vi "RTM - Add Packet.vi"() -> ()   [LabVIEW 2019, in "UDP-Custom-Device System Explorer.lvlib"]
uses:
  UDP-Custom-Device System Explorer.lvlib
  <vilib>/NI VeriStand/Custom Device Tools/Custom Device Utility Library/Custom Device Utility Library.lvlib
  <vilib>/NI VeriStand/Custom Device API/Custom Device API.lvlib
  Property Accessors/Shared Packet Accessors.lvlib
panel:
  in  "Buffered?":bool
  in  "Cancel Button":bool
  in  "OK Button":bool
  out "New Packet ID":i32
  in  "New Packet Name":string
  in  "Tag":string
  in  "Node Ptr":u64 format="%.0x"
  out "error out":errorcluster
  in  "error in (no error)":errorcluster
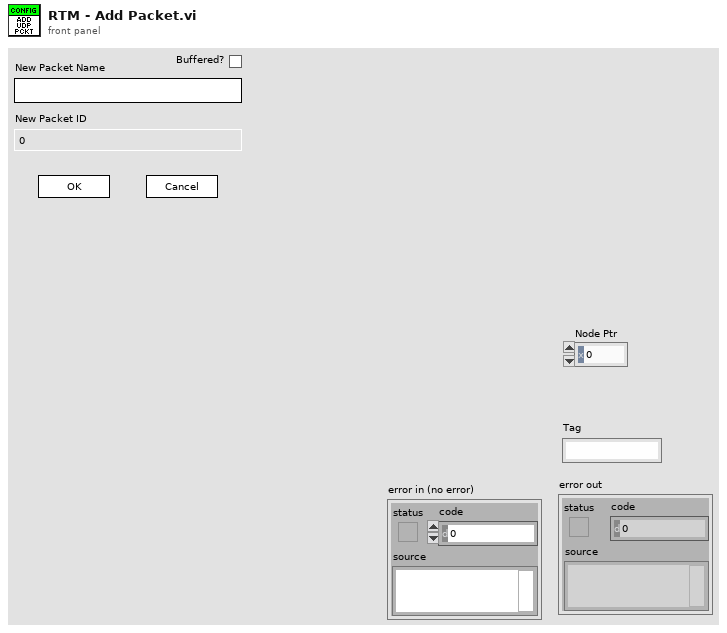
[diagram p1: front panel]
types:
  T1 = enum8{"Enabled", "Disabled", "Disabled and Grayed Out"}
  T2 = enum32{"Invalid", "Standard", "Closed", "Hidden", "Minimized", "Maximized"}
  T3 = typedef "Custom Device API.lvlib/Custom Device Item Ref.ctl" = u64
  T4 = typedef "UDP-Custom-Device System Explorer.lvlib/Packet Type.ctl" = enum16{"Transmit", "Receive", "Buffered Transmit", "Buffered Receive"}
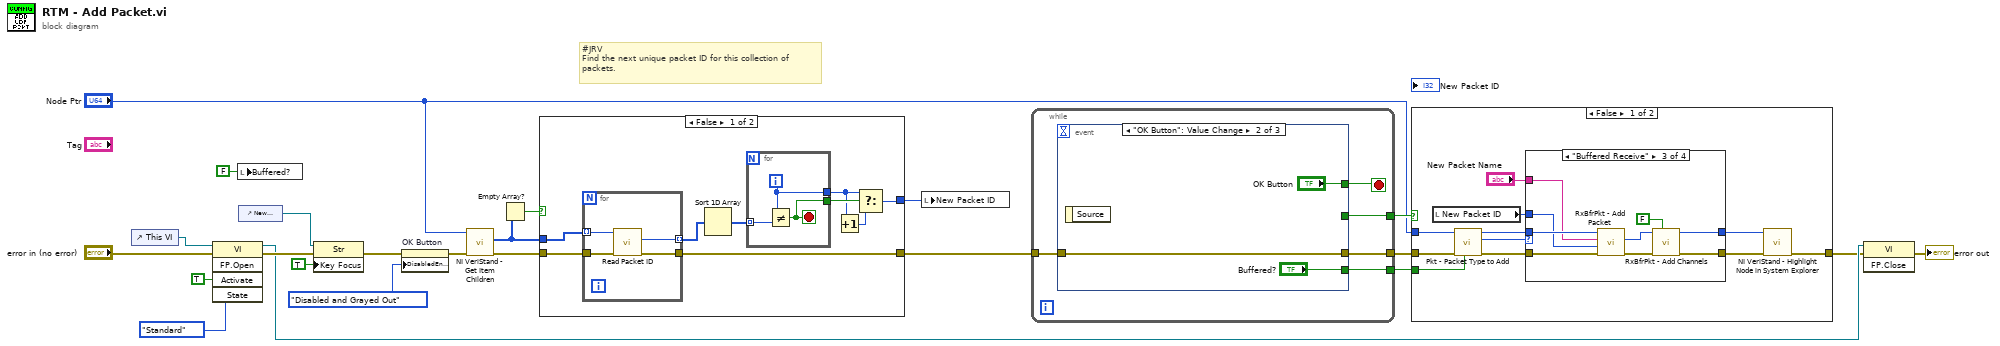
[diagram p0: block diagram]
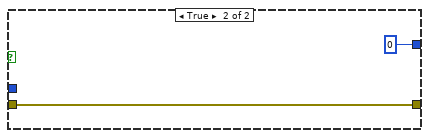
[diagram p2: hidden frame]
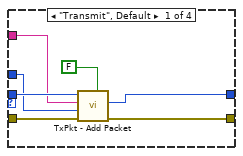
[diagram p3: hidden frame]
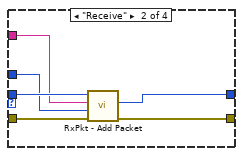
[diagram p4: hidden frame]
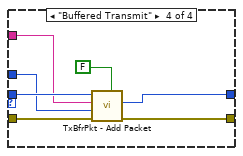
[diagram p5: hidden frame]
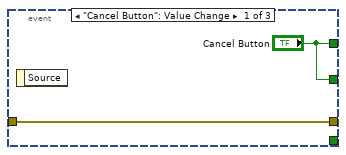
[diagram p7: hidden frame]
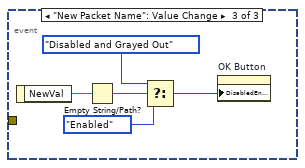
[diagram p8: hidden frame]
diagram:
  # "#JRV\nFind the next unique packet ID for this collection of\npackets."
  n1 = control-ref of="This VI"() -> (w23:refnum<vi>)
  n2 = invoke class="VI" method="FP.Open"(reference=w23, error in="error in (no error)", "Activate"=TRUE ("Activate?"), "State"=T2."Standard") -> (reference out=w15:refnum<vi>, error out=w19:errorcluster)  [unwired: 1 in, 3 out]
  n3 = local write "Buffered?"(FALSE ("Buffered?")) -> ()
  n4 = control-ref of="New Packet Name"() -> (w13:refnum<vi>)
  n5 = property class="Str"(reference=w13, error in=w19, "Key Focus"=TRUE) -> (error out=w4:errorcluster)  [unwired: 1 out]
  n6 = property on="OK Button" class="Bool"(error in=w4, "DisabledEnum"=T1."Disabled and Grayed Out" ("Disabled")) -> (error out=w3:errorcluster)  [unwired: 1 in, 1 out]
  n7 = call <vilib>:"NI VeriStand - Get Item Children.vi"("error in (no error)"=w3, "Item Ref in"="Node Ptr") -> ("error out"=w11:errorcluster, "Child Refs"=w8:T3[])  [unwired: 6 in, 2 out]
  n8 = Empty Array?(array=w8) -> (empty?=w9:bool)
  n9 = case shown="False" w9 {
    tunnel: w11 -> [w31 w41]
    tunnel: [w32 w41] -> w10
    tunnel: w8 -> [w30 _]
    tunnel: [w24 0 ("New Packet ID")] -> w6
    frame False {
      n10 = for {
        tunnel: [w33] -> w32
        tunnel: w31 -> [w35]
        tunnel: w30 -> [w36] mode=indexing
        tunnel: [w34] -> w29 mode=indexing
        n11 = call "Read Packet ID.vi"("error in (no error)"=w35, "Node Ptr"=w36) -> ("error out"=w33:errorcluster, "Packet ID"=w34:i32)  [unwired: 7 in, 1 out]
      }
      n12 = Sort 1D Array(array=w29) -> (sorted array=w28:i32[])
      n13 = for {
        tunnel: w28 -> [w39] mode=indexing
        tunnel: [w38] -> w26
        tunnel: [w37] -> w27
        i -> [w38]
        stop <- w37 stop-if-true
        n14 = Not Equal?(x=w38, y=w39) -> (x != y?=w37:bool)
      }
      n15 = Increment(x=w26) -> (x+1=w25:i32)
      n16 = Select(t=w26, s=w27, f=w25) -> (s? t:f=w24:i32)
    }
    frame True {
    }
  }
  n17 = local write "New Packet ID"(w6) -> ()
  n18 = while {
    tunnel: w10 -> [w45]
    tunnel: [w44] -> w17
    tunnel: [w43] -> w18
    tunnel: [w42] -> w2
    stop <- w46 stop-if-true
    n19 = event shown="[1] \"OK Button\": Value Change" {
      selector: _ -> [_ _ _]
      dyn-events: _ -> [_ _ _]
      timeout: _ -> [_ _ _]
      tunnel: ["Cancel Button" "OK Button" _] -> w46
      tunnel: w45 -> [w48 w49 _]
      tunnel: [w48 w49 _] -> w44
      tunnel: ["Cancel Button" _ _] -> w43
      tunnel: [_ "Buffered?" _] -> w42
      event "Cancel Button": Value Change {
        n20 = event-data() -> ()  [unwired: 1 in, 1 out]
      }
      event "OK Button": Value Change {
        n21 = event-data() -> ()  [unwired: 1 in, 1 out]
      }
      event "New Packet Name": Value Change {
        n22 = event-data() -> ("NewVal"=w56:string)  [unwired: 1 in]
        n23 = Empty String/Path?(string/path=w56) -> (empty?=w55:bool)
        n24 = Select(t=T1."Disabled and Grayed Out" ("Disabled"), s=w55, f=T1."Enabled" ("Disabled")) -> (s? t:f=w52:T1)
        n25 = property on="OK Button" class="Bool"("DisabledEnum"=w52) -> ()  [unwired: 2 in, 2 out]
      }
    }
  }
  n26 = case shown="False" w18 {
    tunnel: w17 -> [w66 w97]
    tunnel: [w59 w97] -> w14
    tunnel: "Node Ptr" -> [w67 _]
    tunnel: w2 -> [w57 _]
    frame False {
      n27 = local read "New Packet ID"() -> (w58:i32)
      n28 = call "Pkt - Packet Type to Add.vi"("Buffered?"=w57, "error in (no error)"=w66, "Item Ref in"=w67) -> ("error out"=w63:errorcluster, "Packet Type"=w65:T4, "Item Ref out"=w64:T3)  [unwired: 6 in]
      n29 = case shown="\"Buffered Receive\"" w65 {
        tunnel: w64 -> [w74 w78 w89 w96]
        tunnel: w63 -> [w73 w80 w86 w95]
        tunnel: "New Packet Name" -> [w72 w77 w88 w93]
        tunnel: w58 -> [w71 w76 w87 w92]
        tunnel: [w70 w79 w81 w94] -> w61
        tunnel: [w69 w75 w84 w91] -> w60
        frame "Transmit", Default {
          n30 = call "TxPkt - Add Packet.vi"("Add Port Channel"=FALSE, "error in (no error)"=w73, "New Packet ID"=w71, "New Packet Name"=w72, "Item Ref in"=w74) -> ("error out"=w70:errorcluster, "New Packet Ref"=w69:T3)  [unwired: 4 in, 1 out]
        }
        frame "Receive" {
          n31 = call "RxPkt - Add Packet.vi"("error in (no error)"=w80, "New Packet ID"=w76, "New Packet Name"=w77, "Item Ref in"=w78) -> ("error out"=w79:errorcluster, "New Packet Ref"=w75:T3)  [unwired: 5 in, 1 out]
        }
        frame "Buffered Receive" {
          n32 = call "RxBfrPkt - Add Packet.vi"("error in (no error)"=w86, "New Packet ID"=w87, "New Packet Name"=w88, "Item Ref in"=w89) -> ("error out"=w82:errorcluster, "New Packet Ref"=w85:T3)  [unwired: 5 in, 1 out]
          n33 = call "RxBfrPkt - Add Channels.vi"("Ext Buffer?"=FALSE, "error in (no error)"=w82, "Node Ptr"=w85) -> ("error out"=w81:errorcluster, "Node Ptr out"=w84:T3)  [unwired: 7 in]
        }
        frame "Buffered Transmit" {
          n34 = call "TxBfrPkt - Add Packet.vi"("Add Port Channel?"=FALSE, "error in (no error)"=w95, "New Packet ID"=w92, "New Packet Name"=w93, "Item Ref in"=w96) -> ("error out"=w94:errorcluster, "New Packet Ref"=w91:T3)  [unwired: 4 in, 1 out]
        }
      }
      n35 = call <vilib>:"NI VeriStand - Highlight Node in System Explorer.vi"("error in (no error)"=w61, "Item Ref in"=w60) -> ("error out"=w59:errorcluster)  [unwired: 8 in, 1 out]
    }
    frame True {
    }
  }
  n36 = invoke class="VI" method="FP.Close"(reference=w15, error in=w14) -> (error out=→"error out":errorcluster)  [unwired: 1 in, 2 out]
